vi "Read Execution time.vi"(8 "error in (no error)":errorcluster, 11 "Report In":refnum<class "Test Report.lvclass">) -> (0 "error out":errorcluster, 1 "Execution time string":string, 2 "Execution time":dbl, 3 "Report Out":refnum<class "Test Report.lvclass">)   [LabVIEW 2020, in "Test Report.lvclass"]
uses:
  Test Report.lvclass
  Test Report.lvclass/Test Report.ctl
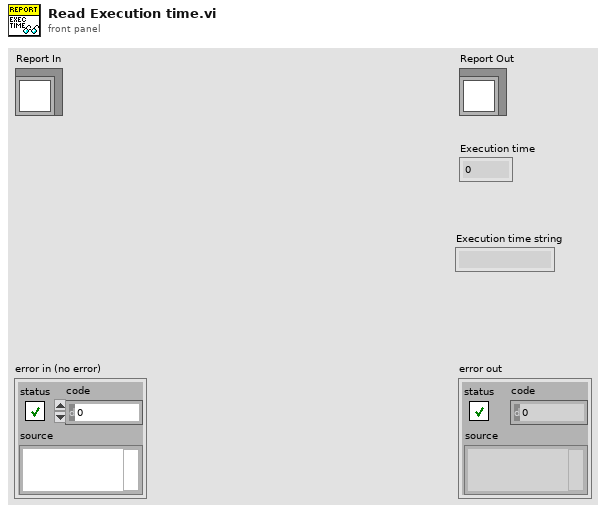
[diagram p1: front panel]
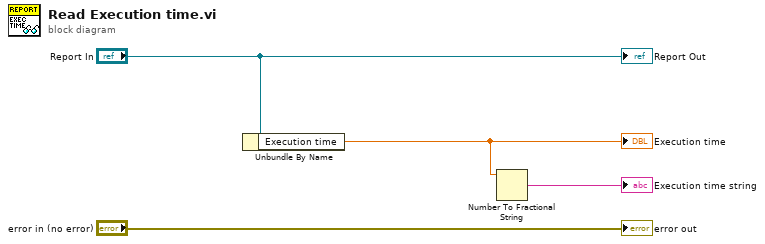
[diagram p0: block diagram]
diagram:
  n1 = Unbundle By Name("Report In") -> ("Execution time"=w2:dbl)
  "Execution time" <- w2
  n2 = Number To Fractional String(number=w2) -> (F-format string=→"Execution time string":string)  [unwired: 3 in]
  "error out" <- "error in (no error)"
  "Report Out" <- "Report In"
